vi "test knight.vi"() -> ()   [LabVIEW 2016]
uses:
  Position/Position.lvclass
  Board/Board.lvclass
  typedef/File.ctl
  Chesslib.lvlib
  typedef/Rank.ctl
  typedef/Square.ctl
  Pieces/Piece/Piece.lvclass
  typedef/Piece type.ctl
  typedef/Color.ctl
  Moves/Move/Move.lvclass
panel:
  in  "Knight":T1={"File"=enum."h", "Rank"=enum."8"}
  out "Array":T1[](array[typedef])
  out "size(s)":i32
  out "Moves":refnum<class "Move.lvclass">[](array[class])
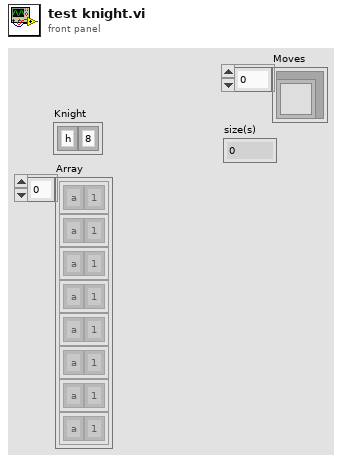
[diagram p1: front panel]
types:
  T1 = typedef "Chesslib.lvlib/Square.ctl" = cluster{"File":T2, "Rank":T3}
  T2 = typedef "Chesslib.lvlib/File.ctl" = enum8{"a", "b", "c", "d", "e", "f", "g", "h"}
  T3 = typedef "Chesslib.lvlib/Rank.ctl" = enum8{"1", "2", "3", "4", "5", "6", "7", "8"}
  T4 = typedef "Chesslib.lvlib/Color.ctl" = enum16{"Light", "Dark"}
  T5 = typedef "Chesslib.lvlib/Piece type.ctl" = enum16{"Pawn", "Bishop", "Knight", "Rook", "Queen", "King"}
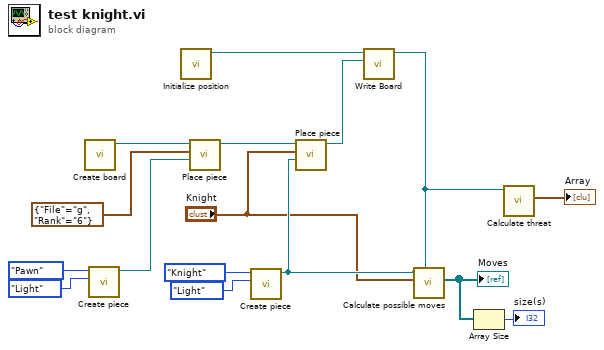
[diagram p0: block diagram]
diagram:
  n1 = call "Create board.vi"() -> ("Empty board"=w15:refnum<class "Board.lvclass">)  [unwired: 11 in]
  n2 = call "Create piece.vi"("Piece color"=Color."Light", "Piece type"=Piece_type."Pawn") -> ("Piece out"=w5:refnum<class "Piece.lvclass">)  [unwired: 9 in]
  n3 = call "Initialize position.vi"() -> ("Position out"=w16:refnum<class "Position.lvclass">)  [unwired: 10 in, 1 out]
  n4 = call "Place piece.vi"("Piece"=w5, "Square"=T1 {"File"=enum."g", "Rank"=enum."6"}, "Board in"=w15) -> ("Board out"=w8:refnum<class "Board.lvclass">)  [unwired: 6 in, 2 out]
  n5 = call "Create piece.vi"("Piece color"=Color."Light", "Piece type"=Piece_type."Knight") -> ("Piece out"=w11:refnum<class "Piece.lvclass">)  [unwired: 9 in]
  n6 = call "Place piece.vi"("Piece"=w11, "Square"="Knight", "Board in"=w8) -> ("Board out"=w12:refnum<class "Board.lvclass">)  [unwired: 6 in, 2 out]
  n7 = call "Write Board.vi"("Board"=w12, "Position in"=w16) -> ("Position out"=w2:refnum<class "Position.lvclass">)  [unwired: 9 in]
  n8 = call-dynamic "Calculate possible moves.vi"("Position"=w2, "Source"="Knight", "Piece in"=w11) -> ("Moves"=w3:refnum<class "Move.lvclass">[])  [unwired: 6 in, 2 out]
  "Moves" <- w3
  n9 = Array Size(array=w3) -> (size(s)=→"size(s)":i32)
  n10 = call "Calculate threat.vi"("Position in"=w2) -> ("Threatened squares"=→"Array":T1[])  [unwired: 8 in, 2 out]
